vi "Sort Indices into Groups.vi"(10 "Indices To Add":T4[](array[typedef]), 11 "Tags":string[](array[string])) -> (2 "Group Initialization Set":T1[](array[typedef]))   [LabVIEW 2020, in "Current Value Table(Rebuild).lvlib"]
doc: "This VI takes a set of indices (data type+index) and sorts them by data type into groups (data type+indices)."
uses:
  Current Value Table(Rebuild).lvlib
  Type Defs/Index Types.ctl
  Type Defs/Data Types.ctl
  Type Defs/Group Initialization set.ctl
  Type Defs/Typed Index Set.ctl
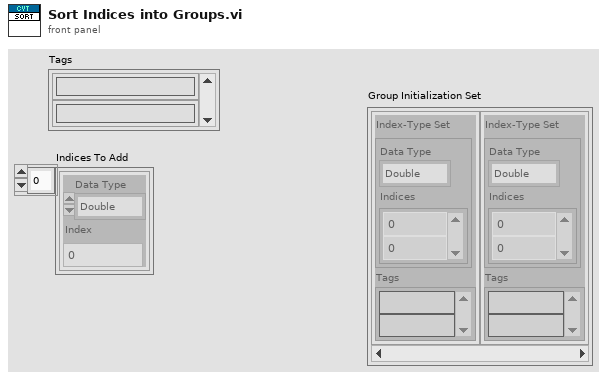
[diagram p1: front panel]
types:
  T1 = typedef "Current Value Table(Rebuild).lvlib/Group Initialization set.ctl" = cluster{"Index-Type Set":T2, "Tags":string[]}
  T2 = typedef "Current Value Table(Rebuild).lvlib/Typed Index Set.ctl" = cluster{"Data Type":T3, "Indices":i32[]}
  T3 = typedef "Current Value Table(Rebuild).lvlib/Data Types.ctl" = enum16{"Double", "Single", "I64", "I32", "I16", "I8", "U64", "U32", "U16", "U8", "String", "Boolean", "Array of U8", "Array of U16", "Array of U32", "Array of U64", "Array of I64", "Array of I32", "Array of I16", "Array of I8", "Array of Double", "Array of Single", "Array of Boolean", "Array of String"}
  T4 = typedef "Current Value Table(Rebuild).lvlib/Index Types.ctl" = cluster{"Data Type":T3, "Index":i32}
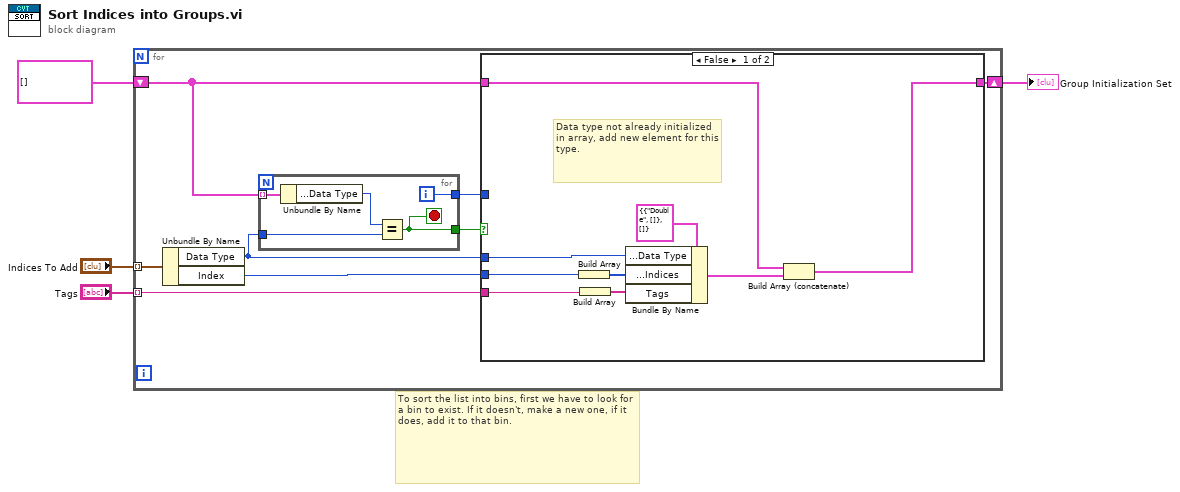
[diagram p0: block diagram]
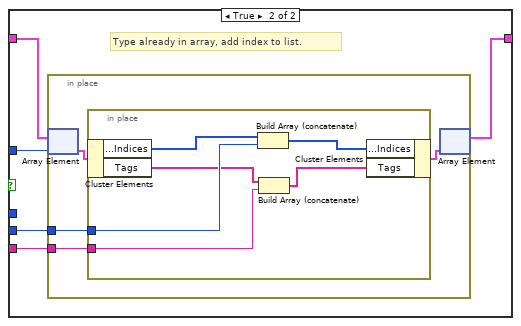
[diagram p2: hidden frame]
diagram:
  # "To sort the list into bins, first we have to look for a bin to exist. If it doesn't, make a new one, if it does, add it to that bin."
  n1 = for {
    tunnel: "Indices To Add" -> [w12] mode=indexing
    shift-right: [w8] -> w2
    shift-left: T1[] [] ("Group Initialization Set") -> [w10]
    tunnel: "Tags" -> [w5] mode=indexing
    n2 = Unbundle By Name(w12) -> ("Data Type"=w6:T3, "Index"=w7:i32)
    n3 = for {
      tunnel: w10 -> [w41] mode=indexing
      tunnel: w6 -> [w39]
      tunnel: [w38] -> w11
      tunnel: [w37] -> w9
      i -> [w37]
      stop <- w38 stop-if-true
      n4 = Unbundle By Name(w41) -> ("Index-Type Set.Data Type"=w40:T3)
      n5 = Equal?(x=w40, y=w39) -> (x = y?=w38:bool)
    }
    n6 = case shown="False" w11 {
      tunnel: w10 -> [w18 w26]
      tunnel: w9 -> [_ w25]
      tunnel: [w17 w24] -> w8
      tunnel: w7 -> [w21 w23]
      tunnel: w6 -> [w20 _]
      tunnel: w5 -> [w14 w22]
      frame False {
        # "Data type not already initialized in array, add new element for this type."
        n7 = Build Array(w21) -> (w19:i32[])
        n8 = Build Array(w14) -> (w13:string[])
        n9 = Bundle By Name(cluster=T1 {"Index-Type Set"={"Data Type"=enum."Double", "Indices"=[]}, "Tags"=[]} ("Group Initialization"), "Index-Type Set.Data Type"=w20, "Index-Type Set.Indices"=w19, "Tags"=w13) -> (w16:T1)
        n10 = Build Array (concatenate)(w18, w16) -> (w17:T1[])
      }
      frame True {
        # "Type already in array, add index to list."
        n11 = in-place {
          in-place-border: w23 -> [w29]
          in-place-border: w22 -> [w27]
          n12 = in-place-array #1(w26, w25) -> (w30:T1)
          n13 = in-place {
            in-place-border: w29 -> [w36]
            in-place-border: w27 -> [w31]
            n14 = in-place-cluster #2(w30) -> ("Index-Type Set.Indices"=w35:i32[], "Tags"=w32:string[])
            n15 = Build Array (concatenate)(w35, w36) -> (w34:i32[])
            n16 = Build Array (concatenate)(w32, w31) -> (w33:string[])
            n17 = in-place-cluster #2("Index-Type Set.Indices"=w34, "Tags"=w33) -> (w28:T1)
          }
          n18 = in-place-array #1(w28) -> (w24:T1[])  [unwired: 1 out]
        }
      }
    }
  }
  "Group Initialization Set" <- w2
